vi "Creator Alias.vi"(11 "Actor in":refnum<class "Actor.lvclass">) -> (2 "Creator Alias":string)   [LabVIEW 2021, in "jettl.lvlib" / "Actor.lvlib" / "Actor.lvclass"]
uses:
  Actor.lvclass
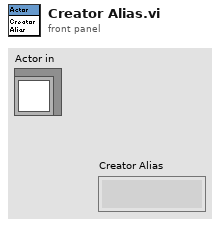
[diagram p1: front panel]
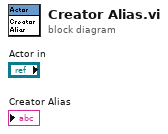
[diagram p0: block diagram]
diagram:
